vi "DAQmx Gated Counter Main.vi"() -> ()   [LabVIEW 2012, in "Waveform.lvclass"]
uses:
  Waveform.lvclass
  <vilib>/DAQmx/create/channels.llb/DAQmx Create Channel (CO-Pulse Generation-Frequency).vi
  <vilib>/DAQmx/configure/timing.llb/DAQmx Timing (Implicit).vi
  <resource>/objmgr/daqmx.rc
panel:
  out "error out 2":errorcluster
  out "error out":errorcluster
  in  "Carrier Frequency":dbl=5500.0
  in  "Gate Frequency":dbl=21.0
  out "CO.Pulse.DutyCyc":dbl
  out "CO.Pulse.Freq":dbl
  in  "Stop":bool
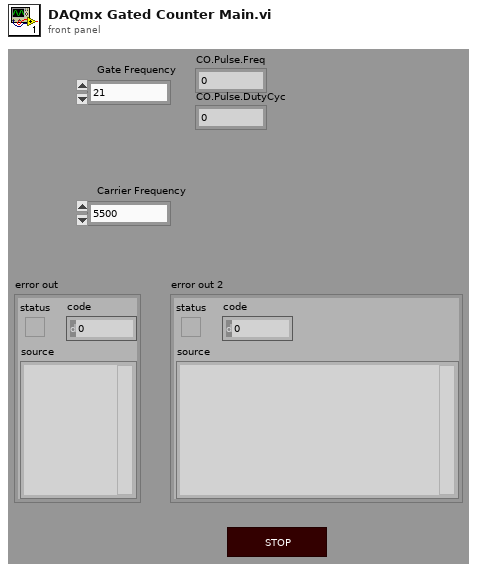
[diagram p1: front panel]
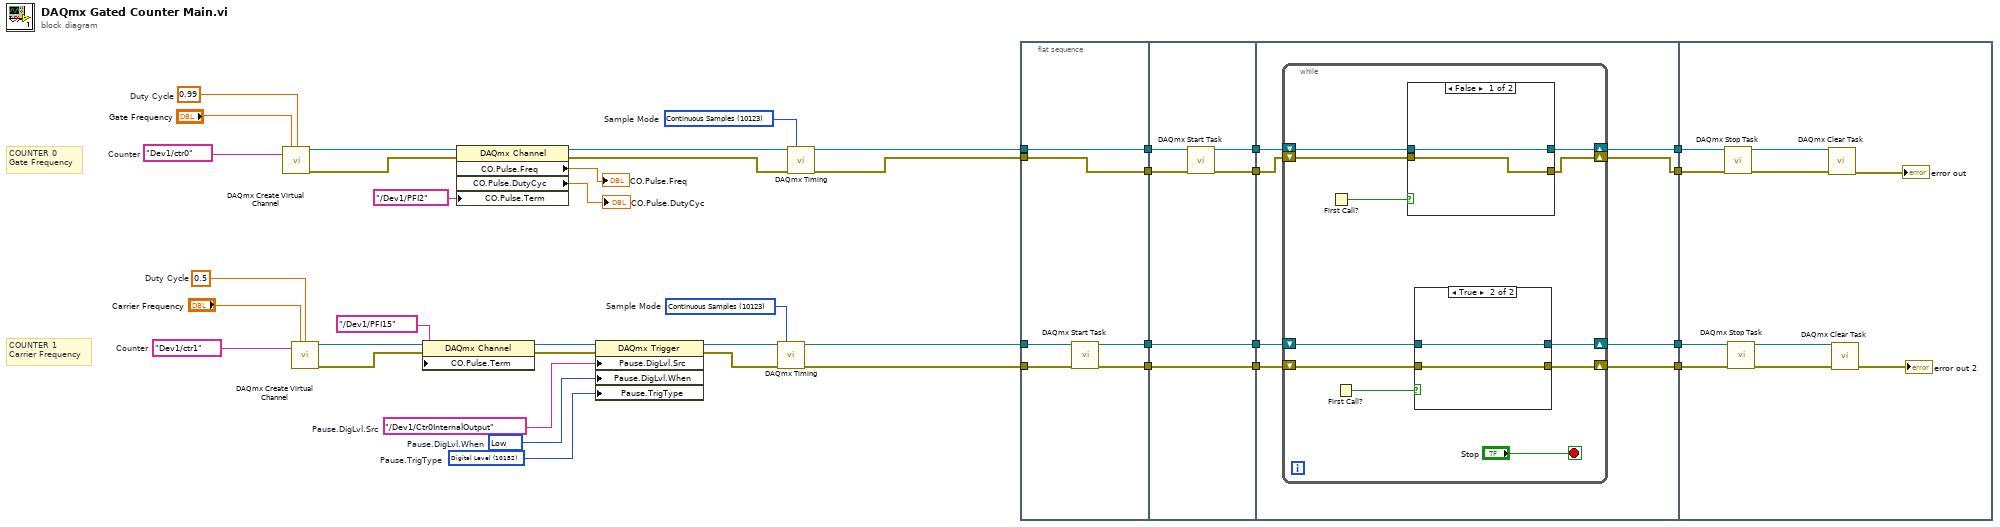
[diagram p0: block diagram]
diagram:
  w19 = 10152 items=["Analog Level"=10101, "Analog Window"=10103, "Digital Level"=10152, "Digital Pattern"=10398, "None"=10230]  # Pause.TrigType
  w20 = 10214 items=["High"=10192, "Low"=10214]  # Pause.DigLvl.When
  w21 = tag "/Dev1/Ctr0InternalOutput"  # Pause.DigLvl.Src
  w30 = 10123 items=["Finite Samples"=10178, "Continuous Samples"=10123, "Hardware Timed Single Point"=12522]  # Sample Mode
  w22 = 0.5  # Duty Cycle
  w31 = tag "Dev1/ctr1"  # Counter
  w34 = 10123 items=["Finite Samples"=10178, "Continuous Samples"=10123, "Hardware Timed Single Point"=12522]  # Sample Mode
  w35 = tag "Dev1/ctr0"  # Counter
  w32 = 0.99  # Duty Cycle
  # "COUNTER 0\nGate Frequency"
  # "COUNTER 1\nCarrier Frequency"
  n1 = call-poly <vilib>:"DAQmx Create Virtual Channel.vi"("frequency"="Gate Frequency", "duty cycle"=w32, "counter"=w35) -> ("task out"=w29:refnum<k21>, "error out"=w28:errorcluster)  [unwired: 11 in]
  n2 = call-poly <vilib>:"DAQmx Create Virtual Channel.vi"("frequency"="Carrier Frequency", "duty cycle"=w22, "counter"=w31) -> ("task out"=w13:refnum<k21>, "error out"=w11:errorcluster)  [unwired: 11 in]
  n3 = property class="DAQmx Channel"(reference=w13, error in=w11, "CO.Pulse.Term"=tag "/Dev1/PFI15") -> (reference out=w12:refnum<k21>, error out=w10:errorcluster)
  n4 = property class="DAQmx Channel"(reference=w29, error in=w28, "CO.Pulse.Term"=tag "/Dev1/PFI2") -> (reference out=w27:refnum<k21>, error out=w26:errorcluster, "CO.Pulse.Freq"=→"CO.Pulse.Freq":dbl, "CO.Pulse.DutyCyc"=→"CO.Pulse.DutyCyc":dbl)
  n5 = property class="DAQmx Trigger"(reference=w12, error in=w10, "Pause.DigLvl.Src"=w21, "Pause.DigLvl.When"=w20, "Pause.TrigType"=w19) -> (reference out=w25:refnum<k21>, error out=w24:errorcluster)
  n6 = call-poly <vilib>:"DAQmx Timing.vi"("task/channels in"=w25, "sample mode"=w30, "error in"=w24) -> ("task out"=w39:refnum<k21>, "error out"=w38:errorcluster)  [unwired: 11 in]
  n7 = call-poly <vilib>:"DAQmx Timing.vi"("task/channels in"=w27, "sample mode"=w34, "error in"=w26) -> ("task out"=w37:refnum<k21>, "error out"=w36:errorcluster)  [unwired: 11 in]
  n8 = flat-sequence {
    tunnel: w36 -> [w46]
    tunnel: w37 -> [w47]
    tunnel: w38 -> [w43]
    tunnel: w39 -> [w45]
    tunnel: [w44] -> w4
    tunnel: [w42] -> w3
    tunnel: [w47] -> w2
    tunnel: [w46] -> w1
    tunnel: [w53] -> w8
    tunnel: [w52] -> w7
    tunnel: [w50] -> w6
    tunnel: [w48] -> w5
    tunnel: w4 -> [w53]
    tunnel: w3 -> [w52]
    tunnel: w2 -> [w51]
    tunnel: w1 -> [w49]
    tunnel: [w57] -> w18
    tunnel: [w56] -> w17
    tunnel: [w55] -> w16
    tunnel: [w54] -> w15
    tunnel: w8 -> [w61]
    tunnel: w7 -> [w60]
    tunnel: w6 -> [w59]
    tunnel: w5 -> [w58]
    tunnel: w18 -> [w87]
    tunnel: w17 -> [w86]
    tunnel: w16 -> [w82]
    tunnel: w15 -> [w81]
    frame #0 {
      n9 = call <vilib>:"DAQmx Start Task.vi"("task/channels in"=w45, "error in"=w43) -> ("task out"=w44:refnum<k21>, "error out"=w42:errorcluster)  [unwired: 12 in]
    }
    frame #1 {
      n10 = call <vilib>:"DAQmx Start Task.vi"("task/channels in"=w51, "error in"=w49) -> ("task out"=w50:refnum<k21>, "error out"=w48:errorcluster)  [unwired: 12 in]
    }
    frame #2 {
      n11 = while {
        shift-right: [w63] -> w55
        shift-left: w61 -> [w69]
        shift-right: [w65] -> w57
        shift-left: w59 -> [w71]
        shift-right: [w64] -> w56
        shift-left: w58 -> [w70]
        shift-right: [w62] -> w54
        shift-left: w60 -> [w68]
        stop <- "Stop" stop-if-true
        n12 = First Call?() -> (First Call?: T/F=w67:bool)
        n13 = First Call?() -> (First Call?: T/F=w66:bool)
        n14 = case shown="False" w67 {
          tunnel: w71 -> [w77 w80]
          tunnel: w70 -> [w78 w79]
          tunnel: [w77 w80] -> w65
          tunnel: [w78 w79] -> w64
          frame False {
          }
          frame True {
          }
        }
        n15 = case shown="True" w66 {
          tunnel: w69 -> [w73 w76]
          tunnel: w68 -> [w74 w75]
          tunnel: [w73 w76] -> w63
          tunnel: [w74 w75] -> w62
          frame False {
          }
          frame True {
          }
        }
      }
    }
    frame #3 {
      n16 = call <vilib>:"DAQmx Stop Task.vi"("task/channels in"=w87, "error in"=w86) -> ("task out"=w90:refnum<k21>, "error out"=w89:errorcluster)  [unwired: 12 in]
      n17 = call <vilib>:"DAQmx Stop Task.vi"("task/channels in"=w82, "error in"=w81) -> ("task out"=w83:refnum<k21>, "error out"=w84:errorcluster)  [unwired: 12 in]
      n18 = call <vilib>:"DAQmx Clear Task.vi"("task in"=w90, "error in"=w89) -> ("error out"=→"error out":errorcluster)  [unwired: 13 in]
      n19 = call <vilib>:"DAQmx Clear Task.vi"("task in"=w83, "error in"=w84) -> ("error out"=→"error out 2":errorcluster)  [unwired: 13 in]
    }
  }
